vi "CheckPosCon.vi"(9 "Sequential Checks":dbl, 10 "WasRight":bool) -> (2 "We made It":bool)   [LabVIEW 2020]
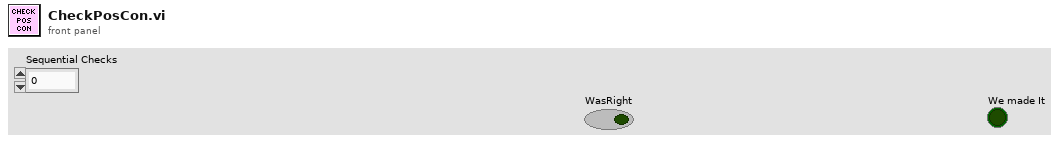
[diagram p1: front panel]
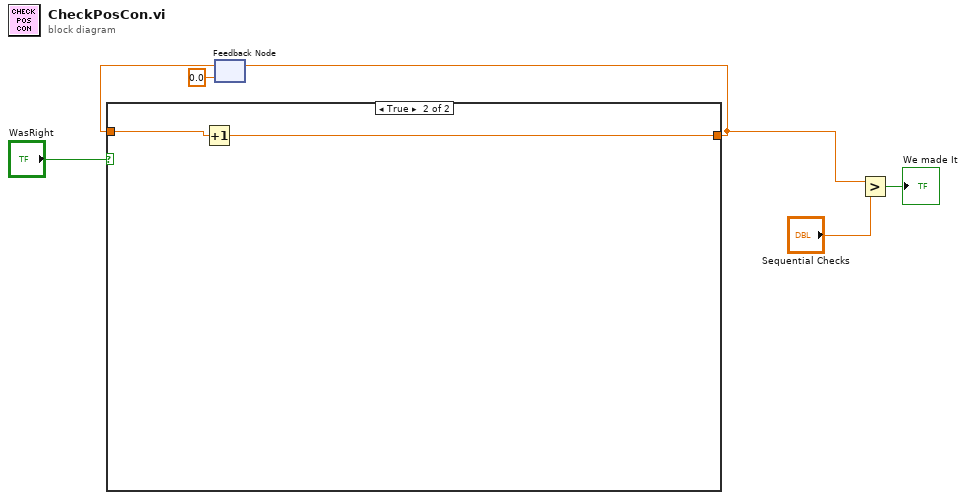
[diagram p0: block diagram]
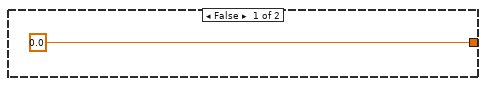
[diagram p2: hidden frame]
diagram:
  n1 = feedback #1(0.0) -> (w6:dbl)
  n2 = case shown="True" "WasRight" {
    tunnel: w6 -> [_ w9]
    tunnel: [0.0 w8] -> w4
    frame False {
    }
    frame True {
      n3 = Increment(x=w9) -> (x+1=w8:dbl)
    }
  }
  n4 = feedback-in #1(w4) -> ()
  n5 = Greater?(x=w4, y="Sequential Checks") -> (0:→"We made It":bool)
